vi "StoreDataArray.vi"(0 "Base path":path=path "D:/CTA/IntegrationBoard/tmp", 1 "X Signal Name":string="Threshold", 2 "Y Signal Name":string="IPR", 3 "Channel number":i32, 4 "Si":string="100mV", 5 "error in":errorcluster, 6 "Save test data":bool, 8 "X Array":dbl[](array[numeric]), 10 "Y Array":dbl[](array[numeric])) -> (19 "error out":errorcluster)   [LabVIEW 2009]
doc: "This VI is specially implemented to store IPR curves into .txt files."
uses:
  <vilib>/express/express signal manip/GetorSetDDTAttributes/Set DDT Attributes/Set DDT Properties.xnode
  <vilib>/express/express shared/transition.llb/Waveform Array To Dynamic.vi
  <vilib>/express/express signal manip/GetorSetDDTAttributes/Set DDT Attributes/SetT0.vi
  <vilib>/express/express shared/transition.llb/Dynamic To Waveform Array.vi
  <vilib>/express/express signal manip/GetorSetDDTAttributes/Shared VIs/XDimension Enum to String.vi
  <vilib>/express/express signal manip/GetorSetDDTAttributes/Shared VIs/XDimension.ctl
  <vilib>/express/express signal manip/GetorSetDDTAttributes/Shared VIs/GetSetShared.lvlib
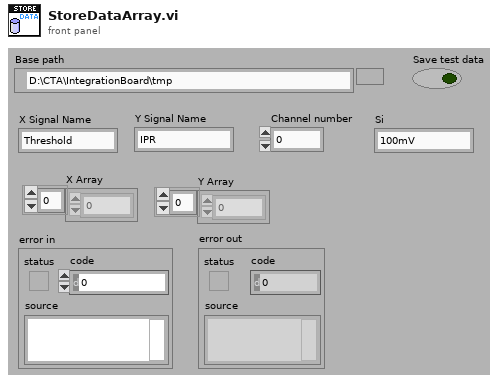
[diagram p1: front panel]
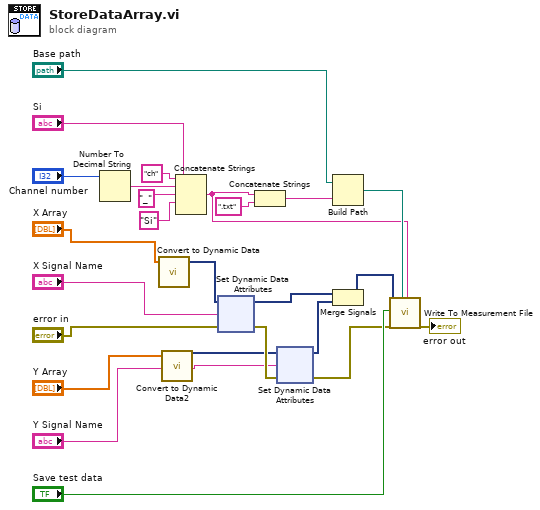
[diagram p0: block diagram]
diagram:
  n1 = Number To Decimal String(number="Channel number") -> (decimal integer string=w17:string)  [unwired: 1 in]
  n2 = call "Convert to Dynamic Data"("Array"="X Array") -> ("Dynamic Data Type"=w10:dynamicdata)  [unwired: 3 in]
  n3 = call "Convert to Dynamic Data2"("Array"="Y Array") -> ("Dynamic Data Type"=w9:dynamicdata)  [unwired: 3 in]
  n4 = Concatenate Strings("ch" ("string"), w17, "_" ("string"), "Si" ("string"), "Si") -> (w2:string)
  n5 = xnode ("Set Dynamic Data Attributes")("Signals In"=w10, "error in"="error in", "Signal Name"="X Signal Name") -> ("Signals Out"=w24:dynamicdata, "error out"=w21:errorcluster)  [unwired: 2 in]
  n6 = Concatenate Strings(w2, ".txt" ("string")) -> (w12:string)
  n7 = xnode ("Set Dynamic Data Attributes")("Signals In"=w9, "error in"=w21, "Signal Name"="Y Signal Name") -> ("Signals Out"=w25:dynamicdata, "error out"=w20:errorcluster)  [unwired: 2 in]
  n8 = Build Path(base path="Base path", name or relative path=w12) -> (appended path=w14:path)
  n9 = Merge Signals(w24, w25) -> (w22:dynamicdata)
  n10 = call "Write To Measurement File"("Signals"=w22, "Enable"="Save test data", "error in (no error)"=w20, "Filename"=w14, "Comment"=w2) -> ("error out"=→"error out":errorcluster)  [unwired: 12 in, 2 out]
